vi "enemy move.vi"(6 "number of enemies":i32, 9 "orientation":dbl[](array[numeric]), 10 "column":dbl[](array[numeric]), 11 "row":dbl[](array[numeric])) -> (1 "orientation":dbl[](array[numeric]), 2 "new column":dbl[](array[numeric]), 3 "new row":dbl[](array[numeric]))   [LabVIEW 2019]
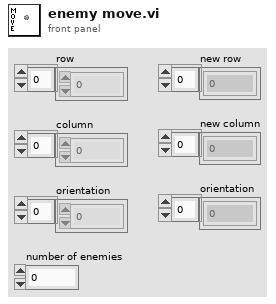
[diagram p1: front panel]
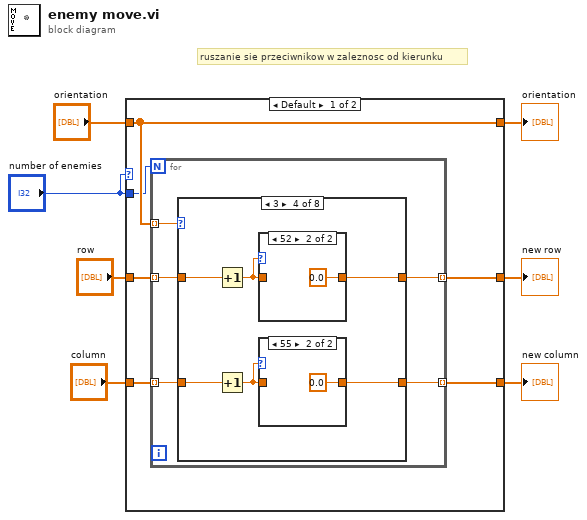
[diagram p0: block diagram]
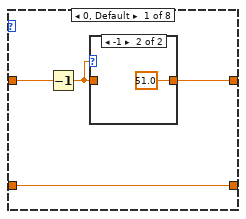
[diagram p2: hidden frame]
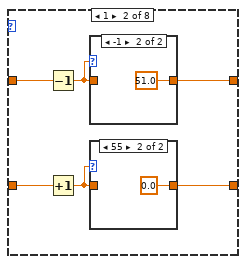
[diagram p4: hidden frame]
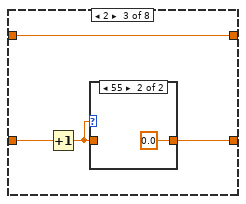
[diagram p7: hidden frame]
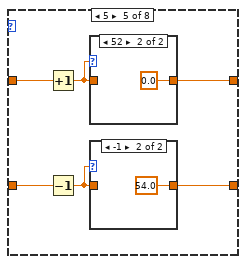
[diagram p11: hidden frame]
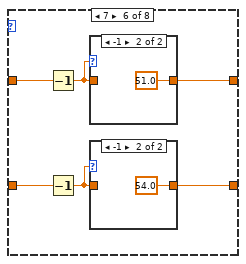
[diagram p14: hidden frame]
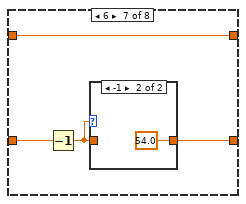
[diagram p17: hidden frame]
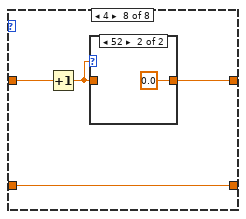
[diagram p19: hidden frame]
diagram:
  # "ruszanie sie przeciwnikow w zaleznosc od kierunku"
  n1 = case shown="Default" "number of enemies" {
    tunnel: "orientation" -> [w13 w83]
    tunnel: "column" -> [w11 w84]
    tunnel: "row" -> [w10 w85]
    tunnel: [w8 w85] -> w4
    tunnel: [w9 w84] -> w5
    tunnel: [w13 w83] -> w6
    tunnel: "number of enemies" -> [w12 _]
    frame Default {
      n2 = for {
        N: w12 -> [_]
        tunnel: w13 -> [w15] mode=indexing
        tunnel: w11 -> [w18] mode=indexing
        tunnel: w10 -> [w17] mode=indexing
        tunnel: [w16] -> w9 mode=indexing
        tunnel: [w14] -> w8 mode=indexing
        n3 = case shown="3" w15 {
          tunnel: w18 -> [w22 w30 w38 w46 w56 w66 w74 w77]
          tunnel: w17 -> [w21 w29 w35 w43 w53 w63 w71 w80]
          tunnel: [w22 w27 w36 w44 w54 w64 w72 w77] -> w16
          tunnel: [w19 w25 w35 w41 w51 w61 w71 w78] -> w14
          frame 0, Default {
            n4 = Decrement(x=w21) -> (x-1=w20:dbl)
            n5 = case shown="-1" w20 {
              tunnel: w20 -> [w23 _]
              tunnel: [w23 51.0] -> w19
              frame Default {
              }
              frame -1 {
              }
            }
          }
          frame 1 {
            n6 = Decrement(x=w29) -> (x-1=w26:dbl)
            n7 = Increment(x=w30) -> (x+1=w28:dbl)
            n8 = case shown="-1" w26 {
              tunnel: w26 -> [w33 _]
              tunnel: [w33 51.0] -> w25
              frame Default {
              }
              frame -1 {
              }
            }
            n9 = case shown="55" w28 {
              tunnel: w28 -> [w31 _]
              tunnel: [w31 0.0] -> w27
              frame Default {
              }
              frame 55 {
              }
            }
          }
          frame 2 {
            n10 = Increment(x=w38) -> (x+1=w37:dbl)
            n11 = case shown="55" w37 {
              tunnel: w37 -> [w39 _]
              tunnel: [w39 0.0] -> w36
              frame Default {
              }
              frame 55 {
              }
            }
          }
          frame 3 {
            n12 = Increment(x=w43) -> (x+1=w42:dbl)
            n13 = Increment(x=w46) -> (x+1=w45:dbl)
            n14 = case shown="52" w42 {
              tunnel: w42 -> [w47 _]
              tunnel: [w47 0.0] -> w41
              frame Default {
              }
              frame 52 {
              }
            }
            n15 = case shown="55" w45 {
              tunnel: w45 -> [w49 _]
              tunnel: [w49 0.0] -> w44
              frame Default {
              }
              frame 55 {
              }
            }
          }
          frame 5 {
            n16 = Increment(x=w53) -> (x+1=w52:dbl)
            n17 = Decrement(x=w56) -> (x-1=w55:dbl)
            n18 = case shown="52" w52 {
              tunnel: w52 -> [w57 _]
              tunnel: [w57 0.0] -> w51
              frame Default {
              }
              frame 52 {
              }
            }
            n19 = case shown="-1" w55 {
              tunnel: w55 -> [w59 _]
              tunnel: [w59 54.0] -> w54
              frame Default {
              }
              frame -1 {
              }
            }
          }
          frame 7 {
            n20 = Decrement(x=w63) -> (x-1=w62:dbl)
            n21 = Decrement(x=w66) -> (x-1=w65:dbl)
            n22 = case shown="-1" w62 {
              tunnel: w62 -> [w67 _]
              tunnel: [w67 51.0] -> w61
              frame Default {
              }
              frame -1 {
              }
            }
            n23 = case shown="-1" w65 {
              tunnel: w65 -> [w69 _]
              tunnel: [w69 54.0] -> w64
              frame Default {
              }
              frame -1 {
              }
            }
          }
          frame 6 {
            n24 = Decrement(x=w74) -> (x-1=w73:dbl)
            n25 = case shown="-1" w73 {
              tunnel: w73 -> [w75 _]
              tunnel: [w75 54.0] -> w72
              frame Default {
              }
              frame -1 {
              }
            }
          }
          frame 4 {
            n26 = Increment(x=w80) -> (x+1=w79:dbl)
            n27 = case shown="52" w79 {
              tunnel: w79 -> [w81 _]
              tunnel: [w81 0.0] -> w78
              frame Default {
              }
              frame 52 {
              }
            }
          }
        }
      }
    }
    frame 0 {
      # "jak byli losowani nowi to \"ruszenie sie\"\nto uznaje jako pojawienie sie"
    }
  }
  "orientation" <- w6
  "new column" <- w5
  "new row" <- w4
